vi "CSDB_Config.get InstanceNames.vi"(2 "ClassName":string, 5 "error in (no error)":errorcluster) -> (16 "InstanceNames":string[](array[string]), 19 "error out":errorcluster)   [LabVIEW 2014, in "CSDB_Config.lvlib"]
doc: "Gets all instances of a class."
uses:
  CSDB_Config.lvlib
  <vilib>/addons/database/_DB Variant To Data/Database Variant To Data.xnode
  <vilib>/addons/database/NI_Database_API.lvlib
  CSDB_Common/CSDB_Common.lvlib
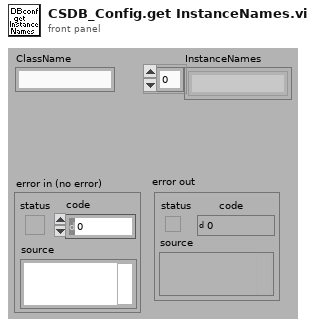
[diagram p1: front panel]
types:
  T1 = typedef "NI_Database_API.lvlib/Conn ObjectReference.ctl" = refnum<k1>
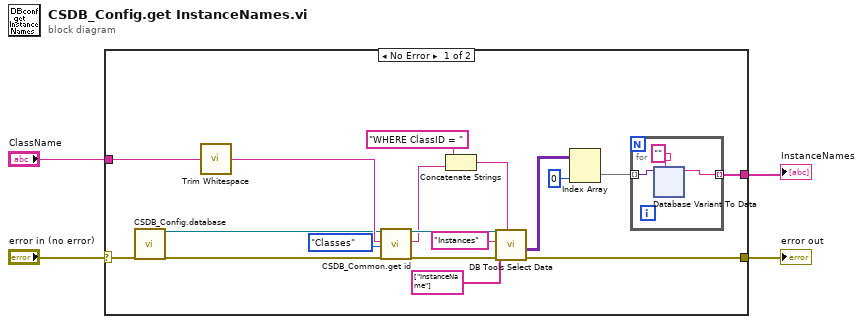
[diagram p0: block diagram]
diagram:
  n1 = case shown="No Error" "error in (no error)" {
    selector: "error in (no error)" -> [w6 w58]
    tunnel: "ClassName" -> [w22 _]
    tunnel: [w11 _] -> w3
    tunnel: [w10 w58] -> w2
    frame No Error {
      n2 = call "CSDB_Config.database.vi"("error in (no error)"=w6) -> ("connectionRef out"=w5:T1, "error out"=w20:errorcluster)  [unwired: 17 in]
      n3 = call <vilib>:"Trim Whitespace.vi"("string"=w22) -> ("trimmed string"=w19:string)  [unwired: 1 in]
      n4 = call "CSDB_Common.get id.vi"("connection reference"=w5, "Class/Attribute/Instance Name"=w19, "Table"=enum16{"Classes", "Attributes", "Instances"}."Classes", "error in (no error)"=w20) -> ("connection reference out"=w18:T1, "ID string"=w16:string, "error out"=w12:errorcluster)  [unwired: 12 in, 1 out]
      n5 = Concatenate Strings("WHERE ClassID = " ("optional clause"), w16) -> (w15:string)
      n6 = call <vilib>:"DB Tools Select Data.vi"("condition"=w15, "error in (no error)"=w12, "columns"=string[] ["InstanceName"], "table"="Instances", "connection reference"=w18) -> ("error out"=w10:errorcluster, "data"=w9:variant[][])  [unwired: 1 in, 1 out]
      n7 = Index Array(array=w9, index (col)=0 ("index (row)")) -> (element=w8:variant[])  [unwired: 1 in]
      n8 = for {
        tunnel: w8 -> [w25] mode=indexing
        tunnel: [w23] -> w11 mode=indexing
        n9 = xnode "Database Variant To Data"("database variant"=w25, "type"="") -> ("data"=w23:string)  [unwired: 1 in, 1 out]
      }
    }
    frame Error {
    }
  }
  "error out" <- w2
  "InstanceNames" <- w3
